vi "Checksum.vi"(1 "Byte2":string="i", 2 "Byte1":string="¢") -> (0 "chaîne":string)   [LabVIEW 2010]
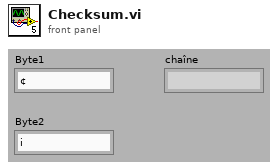
[diagram p1: front panel]
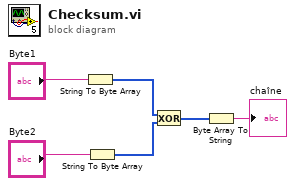
[diagram p0: block diagram]
diagram:
  n1 = String To Byte Array(string="Byte1") -> (unsigned byte array=w3:u8[])
  n2 = String To Byte Array(string="Byte2") -> (unsigned byte array=w4:u8[])
  n3 = Exclusive Or(1:w4, 2:w3) -> (0:w5:u8[])
  n4 = Byte Array To String(unsigned byte array=w5) -> (string=→"chaîne":string)
